vi "test_mode_calculator.vi"(0 "Mode":T2(ring), 1 "T1":dbl min=0.0 format="%.2f", 2 "Delay":dbl min=0.0 format="%.2f", 3 "T2":dbl min=0.0 format="%.2f") -> (6 "Mode parameters":T1 {"Total test time" format="%.2f"; "overlap" format="%.2f"; "Second time test" format="%.2f"; "First time test" format="%.2f"})   [LabVIEW 2015]
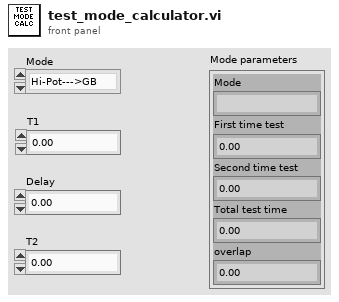
[diagram p1: front panel]
types:
  T1 = cluster{"First time test":dbl, "Second time test":dbl, "overlap":dbl, "Total test time":dbl, "Mode":string}
  T2 = enum16{"Hi-Pot--->GB", "GB--->Hi-Pot", "Hi-Pot only", "GB only"}
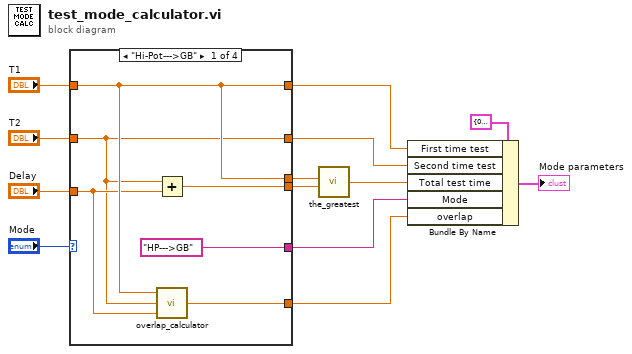
[diagram p0: block diagram]
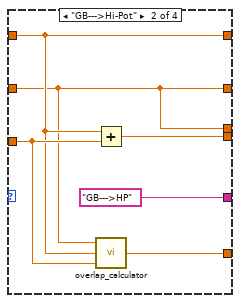
[diagram p2: hidden frame]
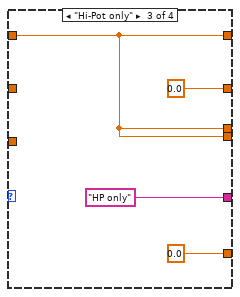
[diagram p3: hidden frame]
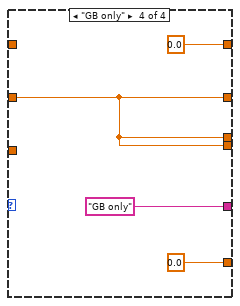
[diagram p4: hidden frame]
diagram:
  n1 = case shown="\"Hi-Pot--->GB\"" "Mode" {
    tunnel: "T1" -> [w16 w21 w27 _]
    tunnel: "T2" -> [w14 w20 _ w31]
    tunnel: "Delay" -> [w15 w22 _ _]
    tunnel: [w19 w25 w27 w31] -> w13
    tunnel: [w16 w20 w27 w31] -> w12
    tunnel: [w16 w21 w27 0.0] -> w5
    tunnel: [w14 w20 0.0 w31] -> w6
    tunnel: ["HP--->GB" "GB--->HP" "HP only" "GB only"] -> w3
    tunnel: [w17 w23 0.0 0.0] -> w2
    frame "Hi-Pot--->GB" {
      n2 = Add(x=w14, y=w15) -> (x+y=w19:dbl)
      n3 = call "overlap_calculator.vi"("T1"=w16, "T2"=w14, "D"=w15) -> ("overlap"=w17:dbl)  [unwired: 4 in]
    }
    frame "GB--->Hi-Pot" {
      n4 = Add(x=w21, y=w22) -> (x+y=w25:dbl)
      n5 = call "overlap_calculator.vi"("T1"=w20, "T2"=w21, "D"=w22) -> ("overlap"=w23:dbl)  [unwired: 4 in]
    }
    frame "Hi-Pot only" {
    }
    frame "GB only" {
    }
  }
  n6 = call "the_greatest.vi"("A"=w12, "B"=w13) -> ("max"=w4:dbl)  [unwired: 6 in]
  n7 = Bundle By Name(cluster=T1 {"First time test"=0.0, "Second time test"=0.0, "overlap"=0.0, "Total test time"=0.0, "Mode"=""} ("Mode parameters"), "First time test"=w5, "Second time test"=w6, "Total test time"=w4, "Mode"=w3, "overlap"=w2) -> (→"Mode parameters":T1)
